vi "Dmux8Way.vi"(7 "in":bool, 12 "sel":bool[](array[boolean])=[FALSE, FALSE, FALSE]) -> (2 "a":bool, 3 "b":bool, 4 "c":bool, 6 "d":bool, 8 "e":bool, 10 "f":bool, 14 "h":bool, 15 "g":bool)   [LabVIEW 2014]
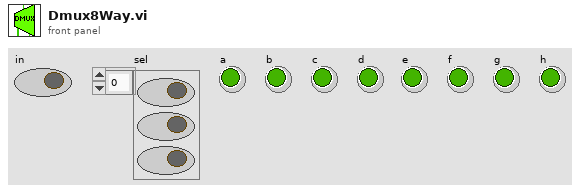
[diagram p1: front panel]
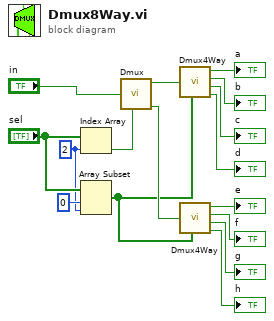
[diagram p0: block diagram]
diagram:
  w1 = 2 ("index")
  n1 = Index Array(array="sel", index=w1) -> (element=w8:bool)
  n2 = Array Subset(array="sel", index=0, length=w1) -> (w3:bool[])
  n3 = call "Dmux.vi"("in"="in", "sel"=w8) -> ("a"=w6:bool, "b"=w5:bool)  [unwired: 7 in]
  n4 = call "Dmux4Way.vi"("in"=w6, "sel"=w3) -> ("a"=→"a":bool, "b"=→"b":bool, "c"=→"c":bool, "d"=→"d":bool)  [unwired: 5 in]
  n5 = call "Dmux4Way.vi"("in"=w5, "sel"=w3) -> ("a"=→"e":bool, "b"=→"f":bool, "c"=→"g":bool, "d"=→"h":bool)  [unwired: 5 in]
